vi "Create TestCase Template Instance.vi"(8 "error in":errorcluster, 11 "Application Ref (This Application)":refnum<vi>) -> (0 "error out":errorcluster, 3 "Application Ref":refnum<vi>)   [LabVIEW 2011, in "VITesterUtilities.lvlib"]
uses:
  Libraries/VITesterUtilities.lvlib
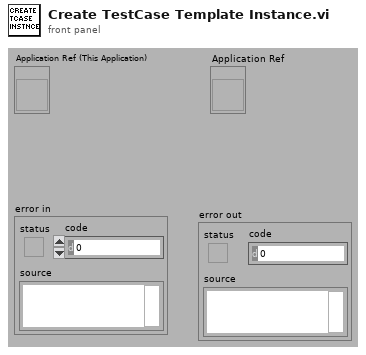
[diagram p1: front panel]
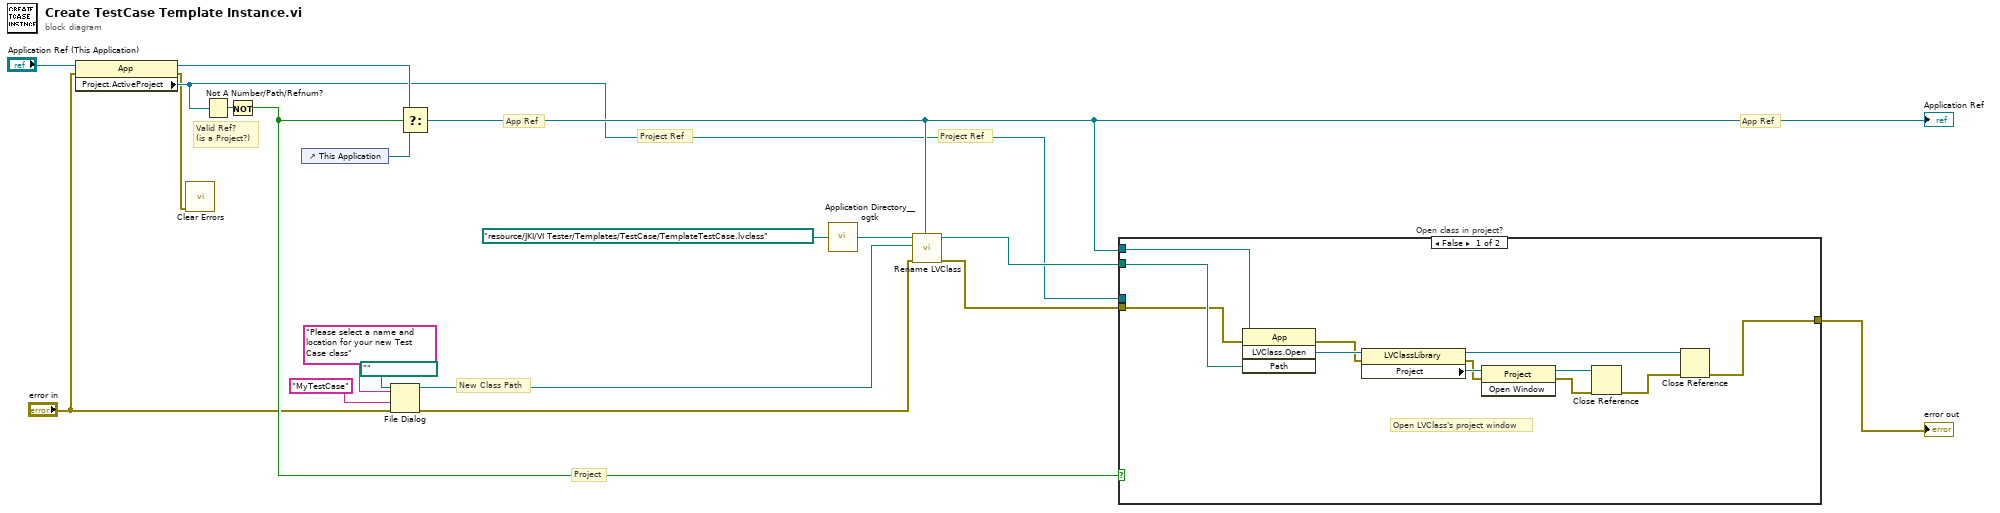
[diagram p0: block diagram]
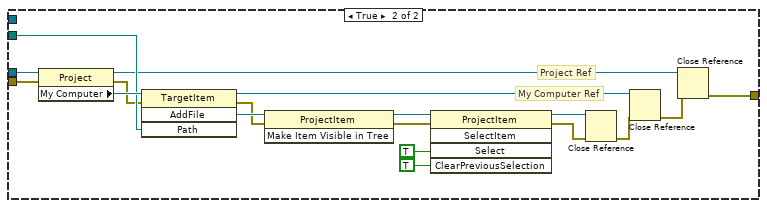
[diagram p2: hidden frame]
diagram:
  # "Project Ref"
  # "App Ref"
  # "Valid Ref?\n(is a Project?)"
  # "Project"
  # "Project Ref"
  # "App Ref"
  # "New Class Path"
  n1 = property class="App"(reference="Application Ref (This Application)", error in="error in") -> (reference out=w10:refnum<vi>, error out=w5:errorcluster, "Project.ActiveProject"=w6:refnum<vi>)
  n2 = call <vilib>:"Clear Errors.vi"("error in (no error)"=w5) -> ()  [unwired: 6 in, 1 out]
  n3 = Not A Number/Path/Refnum?(number/path/refnum=w6) -> (NaN/Path/Refnum?=w12:bool)
  n4 = Not(x=w12) -> (.not. x?=w7:bool)
  n5 = control-ref of="This Application"() -> (w11:refnum<vi>)
  n6 = File Dialog(7:"Please select a name and location for your new Test Case class" ("prompt"), 8:"error in", 9:"MyTestCase" ("default name"), 11:path "" ("start path")) -> (0:w1:errorcluster, 3:w3:path)  [unwired: 3 in, 2 out]
  n7 = Select(t=w10, s=w7, f=w11) -> (s? t:f=w8:refnum<vi>)
  "Application Ref" <- w8
  n8 = call <userlib>:"Application Directory__ogtk.vi"("Relative path (.)"=path "resource/JKI/VI Tester/Templates/TestCase/TemplateTestCase.lvclass") -> ("Application Directory (+ Relative)"=w2:path)
  n9 = call "Rename LVClass.vi"("App reference"=w8, "error in (no error)"=w1, "Destination Path"=w3, "Source Class Path"=w2) -> ("error out"=w17:errorcluster, "Updated LVClass Path"=w16:path)  [unwired: 6 in]
  n10 = case "Open class in project?" shown="False" w7 {
    tunnel: w16 -> [w29 w48]
    tunnel: w17 -> [w28 w46]
    tunnel: [w26 w41] -> w18
    tunnel: w6 -> [_ w32]
    tunnel: w8 -> [w22 _]
    frame False {
      # "Open LVClass's project window"
      n11 = invoke class="App" method="LVClass.Open"(reference=w22, error in=w28, "Path"=w29) -> (error out=w30:errorcluster, "LVClass.Open"=w31:refnum<vi>)  [unwired: 1 in, 2 out]
      n12 = property class="LVClassLibrary"(reference=w31, error in=w30) -> (reference out=w27:refnum<vi>, error out=w24:errorcluster, "Project"=w25:refnum<vi>)
      n13 = invoke class="Project" method="Open Window"(reference=w25, error in=w24) -> (reference out=w23:refnum<vi>, error out=w21:errorcluster)  [unwired: 1 in, 1 out]
      n14 = Close Reference(reference=w23, error in (no error)=w21) -> (error out=w20:errorcluster)
      n15 = Close Reference(reference=w27, error in (no error)=w20) -> (error out=w26:errorcluster)
    }
    frame True {
      # "My Computer Ref"
      # "Project Ref"
      n16 = property class="Project"(reference=w32, error in=w46) -> (reference out=w43:refnum<vi>, error out=w47:errorcluster, "My Computer"=w49:refnum<vi>)
      n17 = invoke class="TargetItem" method="AddFile"(reference=w49, error in=w47, "Path"=w48) -> (reference out=w44:refnum<vi>, error out=w39:errorcluster, "AddFile"=w40:refnum<vi>)  [unwired: 1 in, 1 out]
      n18 = invoke class="ProjectItem" method="Make Item Visible in Tree"(reference=w40, error in=w39) -> (reference out=w36:refnum<vi>, error out=w38:errorcluster)  [unwired: 1 in, 1 out]
      n19 = invoke class="ProjectItem" method="SelectItem"(reference=w36, error in=w38, "Select"=TRUE, "ClearPreviousSelection"=TRUE) -> (reference out=w35:refnum<vi>, error out=w37:errorcluster)  [unwired: 1 in, 3 out]
      n20 = Close Reference(reference=w35, error in (no error)=w37) -> (error out=w45:errorcluster)
      n21 = Close Reference(reference=w44, error in (no error)=w45) -> (error out=w42:errorcluster)
      n22 = Close Reference(reference=w43, error in (no error)=w42) -> (error out=w41:errorcluster)
    }
  }
  "error out" <- w18
